vi "Generate Acoustic Sine Signal.vi"(0 "Sampling Rate":dbl, 1 "Maximum No. of Samples Allowed":i32=65536, 5 "Frequency":dbl, 7 "Sine wave amplitude":dbl=0.01 format="%#_13g", 11 "error in (no error)":errorcluster) -> (4 "waveform":waveform(dbl), 6 "Actual Frequency":dbl, 15 "error out":errorcluster)   [LabVIEW 2020]
doc: "Generate Acoustic Sine Signal VI checks whether the requested frequency can be produced for the given sample rate and outputs Whole Sine waveform of integral multiple of samples for rounded off Sine frequency."
uses:
  <vilib>/Analysis/NI_AALBase.lvlib
  <vilib>/gmath/NI_Gmath.lvlib
  <vilib>/measure/NI_MABase.lvlib
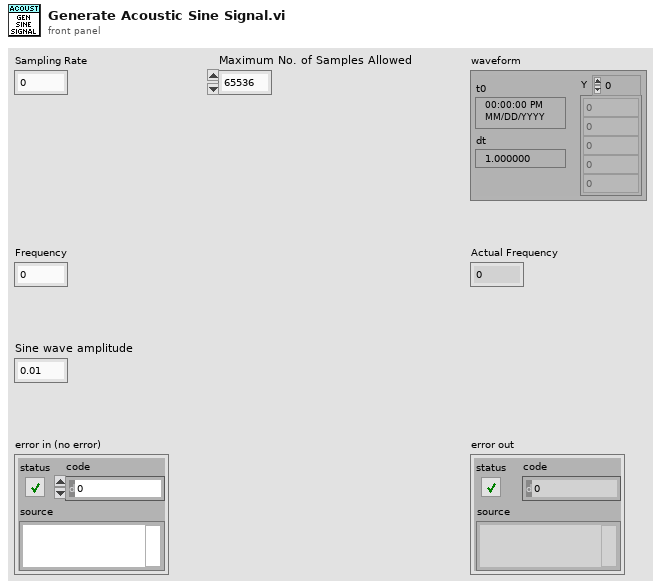
[diagram p1: front panel]
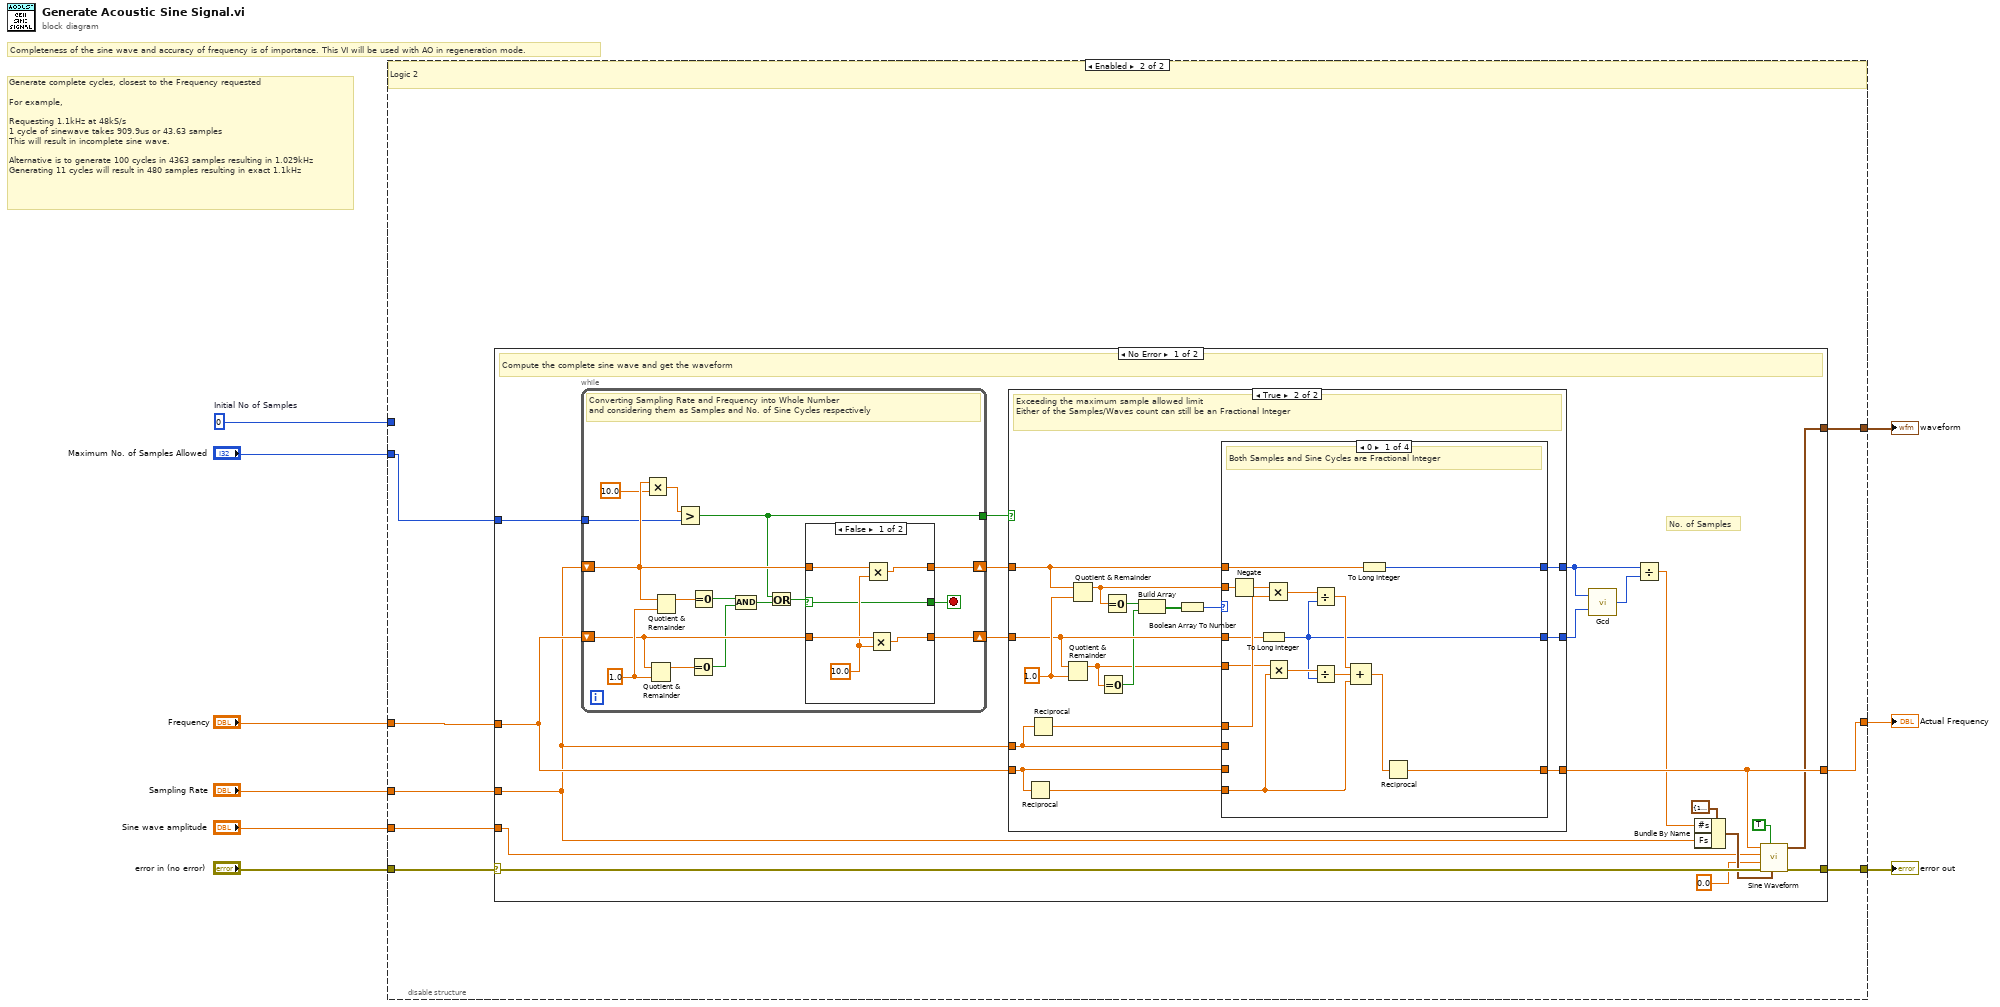
[diagram p0: block diagram]
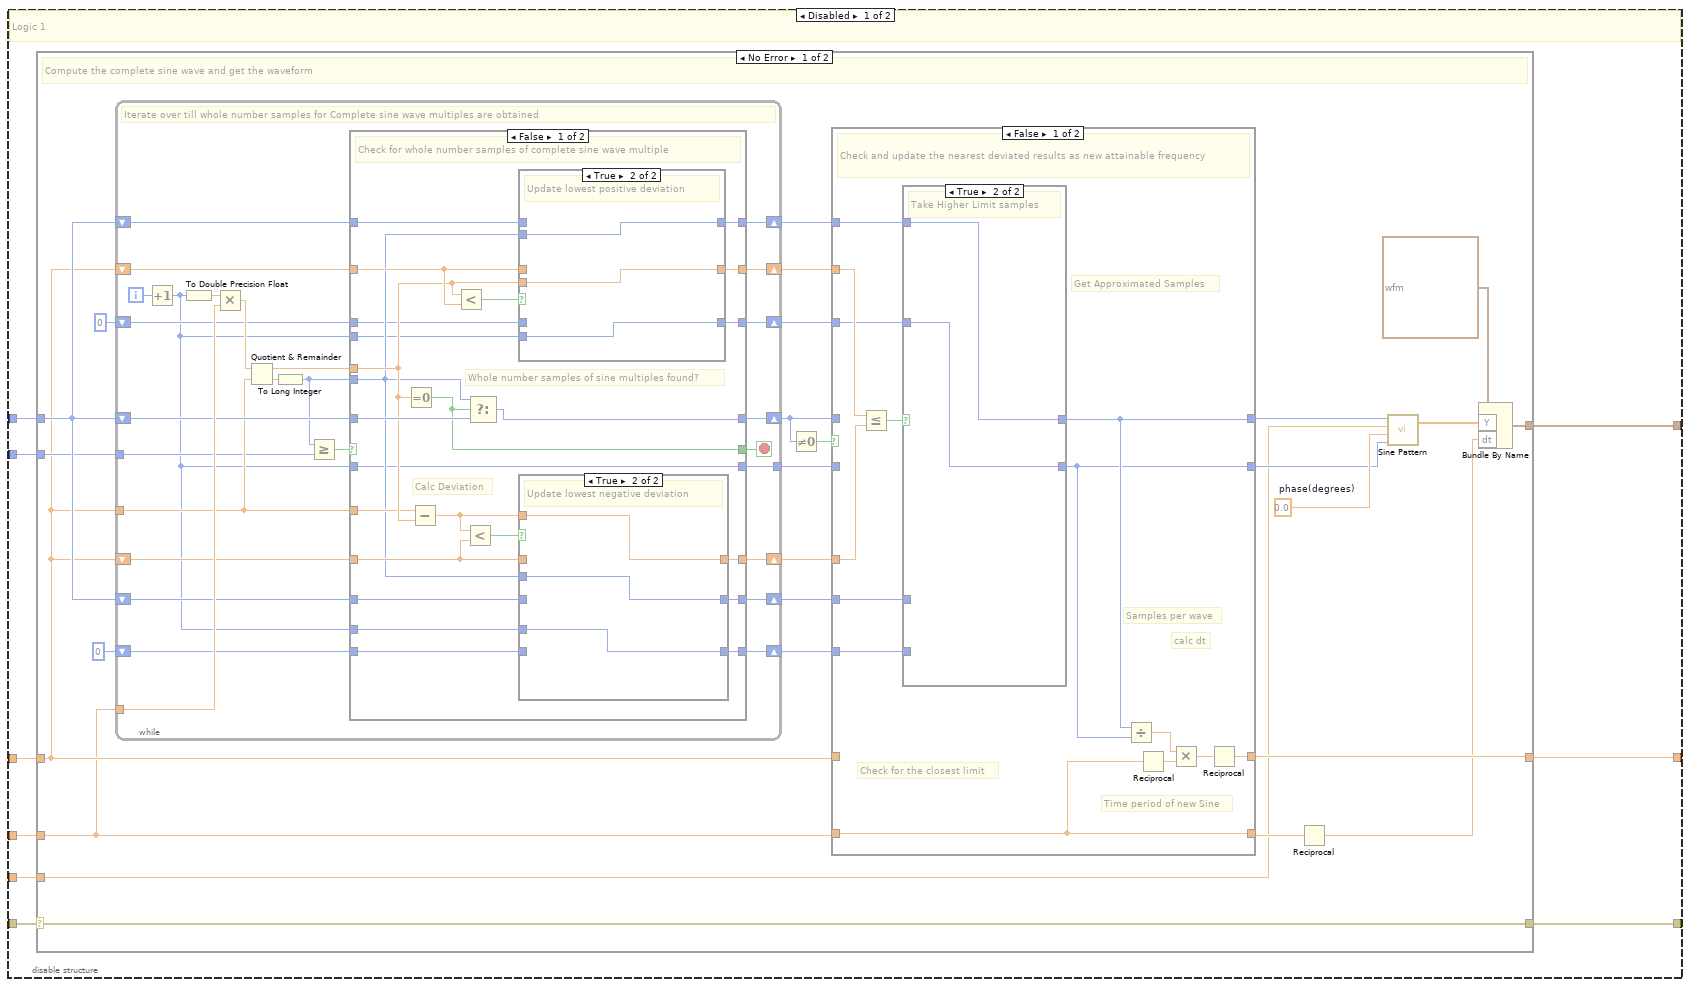
[diagram p2: hidden frame]
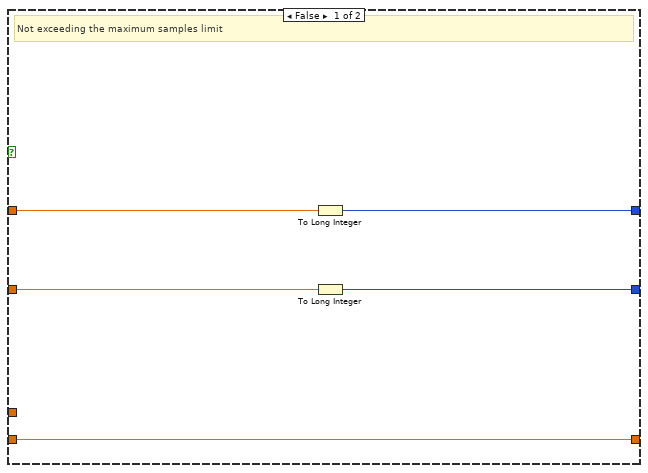
[diagram p9: hidden frame]
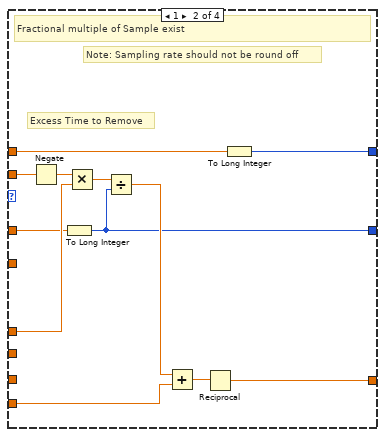
[diagram p10: hidden frame]
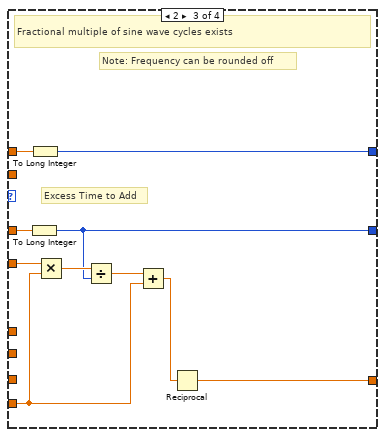
[diagram p11: hidden frame]
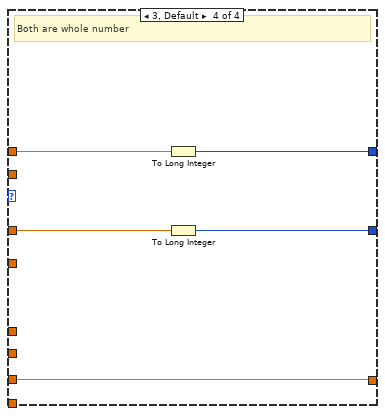
[diagram p12: hidden frame]
diagram:
  w9 = 0  # Initial No of Samples
  # "Completeness of the sine wave and accuracy of frequency is of importance. This VI will be used with AO in regeneration mode."
  # "Generate complete cycles, closest to the Frequency requested\n\nFor example,\n\nRequesting 1.1kHz at 48kS/s\n1 cycle of sinewave takes 909.9us or 43.63 samples\nThis will result in incomplete sine wave. \n\nAlternative is to generate 100 cycles in 4363 samples resulting in 1.029kHz \nGenerating 11 cycles will result in 480 samples resulting in exact 1.1kHz"
  n1 = disable-structure shown="Enabled" {
    disable-tunnel: w9 -> [w18 _]
    disable-tunnel: "Maximum No. of Samples Allowed" -> [w17 w147]
    disable-tunnel: "Frequency" -> [w16 w145]
    disable-tunnel: [w15 w141] -> w6
    disable-tunnel: "Sampling Rate" -> [w14 w146]
    disable-tunnel: [w13 w140] -> w4
    disable-tunnel: "error in (no error)" -> [w12 w144]
    disable-tunnel: [w11 w142] -> w2
    disable-tunnel: "Sine wave amplitude" -> [w10 w143]
    frame Disabled {
      # "Logic 1"
      n2 = case shown="No Error" w12 {
        selector: w12 -> [w25 w139]
        tunnel: w18 -> [w44 _]
        tunnel: w17 -> [w43 _]
        tunnel: w16 -> [w37 _]
        tunnel: [w36 _] -> w15
        tunnel: w14 -> [w35 _]
        tunnel: [w26 _] -> w13
        tunnel: [w25 w139] -> w11
        tunnel: w10 -> [w24 _]
        frame No Error {
          w32 = 0.0  # phase(degrees)
          # "Compute the complete sine wave and get the waveform"
          n3 = while {
            tunnel: w35 -> [w69]
            tunnel: w37 -> [w60]
            shift-right: [w65] -> w41
            shift-left: w44 -> [w64]
            shift-right: [w66] -> w39
            shift-left: w37 -> [w67]
            shift-right: [w62] -> w42
            shift-left: w44 -> [w63]
            shift-right: [w58] -> w38
            shift-left: w37 -> [w59]
            shift-right: [w56] -> w40
            shift-left: w44 -> [w57]
            tunnel: w43 -> [w55]
            tunnel: [w50] -> w34
            shift-right: [w49] -> w19
            shift-left: 0 -> [w48]
            shift-right: [w45] -> w20
            shift-left: 0 ("Initial No of Samples") -> [w47]
            i -> [w71]
            stop <- w51 stop-if-true
            # "Iterate over till whole number samples for Complete sine wave multiples are obtained"
            n4 = Increment(x=w71) -> (x+1=w46:i32)
            n5 = To Double Precision Float(number=w46) -> (double precision float=w70:dbl)
            n6 = Multiply(x=w70, y=w69) -> (x*y=w68:dbl)
            n7 = Quotient & Remainder(x=w68, y=w60) -> (x-y*floor(x/y)=w61:dbl, floor(x/y)=w54:dbl)
            n8 = To Long Integer(number=w54) -> (32bit integer=w53:i32)
            n9 = Greater Or Equal?(x=w53, y=w55) -> (x >= y?=w52:bool)
            n10 = case shown="False" w52 {
              selector: w52 -> [_ w116]
              tunnel: w67 -> [w94 w114]
              tunnel: [w93 w114] -> w66
              tunnel: [w92 w113] -> w65
              tunnel: w64 -> [w91 w113]
              tunnel: w63 -> [w90 w115]
              tunnel: [w89 w115] -> w62
              tunnel: w61 -> [w88 _]
              tunnel: w60 -> [w87 _]
              tunnel: w59 -> [w84 w112]
              tunnel: [w83 w112] -> w58
              tunnel: w57 -> [w82 w111]
              tunnel: [w81 w111] -> w56
              tunnel: w53 -> [w80 _]
              tunnel: [w78 w116] -> w51
              tunnel: w46 -> [w79 w110]
              tunnel: [w79 w110] -> w50
              tunnel: w46 -> [w77 _]
              tunnel: [w76 w109] -> w49
              tunnel: w48 -> [w75 w109]
              tunnel: w47 -> [w74 w108]
              tunnel: w46 -> [w72 _]
              tunnel: [w73 w108] -> w45
              frame False {
                # "Calc Deviation"
                # "Whole number samples of sine multiples found?"
                # "Check for whole number samples of complete sine wave multiple"
                n11 = Equal To 0?(x=w88) -> (x = 0?=w78:bool)
                n12 = Subtract(x=w87, y=w88) -> (x-y=w85:dbl)
                n13 = Less?(x=w88, y=w94) -> (x < y?=w95:bool)
                n14 = Less?(x=w85, y=w84) -> (x < y?=w86:bool)
                n15 = Select(t=w80, s=w78, f=w90) -> (s? t:f=w89:i32)
                n16 = case shown="True" w95 {
                  tunnel: w94 -> [w104 _]
                  tunnel: w88 -> [_ w107]
                  tunnel: [w104 w107] -> w93
                  tunnel: [w103 w106] -> w92
                  tunnel: w91 -> [w103 _]
                  tunnel: w80 -> [_ w106]
                  tunnel: w77 -> [_ w105]
                  tunnel: [w102 w105] -> w76
                  tunnel: w75 -> [w102 _]
                  frame False {
                    # "No Update"
                  }
                  frame True {
                    # "Update lowest positive deviation"
                  }
                }
                n17 = case shown="True" w86 {
                  tunnel: w85 -> [_ w101]
                  tunnel: w84 -> [w98 _]
                  tunnel: [w98 w101] -> w83
                  tunnel: w80 -> [_ w100]
                  tunnel: w82 -> [w97 _]
                  tunnel: [w97 w100] -> w81
                  tunnel: w74 -> [w96 _]
                  tunnel: [w96 w99] -> w73
                  tunnel: w72 -> [_ w99]
                  frame False {
                    # "No Update"
                  }
                  frame True {
                    # "Update lowest negative deviation"
                  }
                }
              }
              frame True {
                # "Maximum sample limit has been reached\nExit the Looping"
              }
            }
          }
          n18 = Not Equal To 0?(x=w42) -> (x != 0?=w23:bool)
          n19 = case shown="False" w23 {
            tunnel: w42 -> [_ w138]
            tunnel: w41 -> [w120 _]
            tunnel: w40 -> [w122 _]
            tunnel: [w118 w138] -> w33
            tunnel: w39 -> [w130 _]
            tunnel: w38 -> [w129 _]
            tunnel: w37 -> [_ w137]
            tunnel: [w126 w137] -> w36
            tunnel: w35 -> [w124 w135]
            tunnel: w34 -> [_ w136]
            tunnel: [w117 w136] -> w31
            tunnel: [w124 w135] -> w28
            tunnel: w20 -> [w121 _]
            tunnel: w19 -> [w119 _]
            frame False {
              # "Time period of new Sine"
              # "calc dt"
              # "Samples per wave"
              # "Get Approximated Samples"
              # "Check for the closest limit"
              # "Check and update the nearest deviated results as new attainable frequency"
              n20 = Less Or Equal?(x=w130, y=w129) -> (x <= y?=w123:bool)
              n21 = case shown="True" w123 {
                tunnel: w122 -> [w132 _]
                tunnel: w121 -> [w131 _]
                tunnel: w120 -> [_ w134]
                tunnel: w119 -> [_ w133]
                tunnel: [w132 w134] -> w118
                tunnel: [w131 w133] -> w117
                frame False {
                  # "Take Lower limit samples"
                }
                frame True {
                  # "Take Higher Limit samples"
                }
              }
              n22 = Divide(x=w118, y=w117) -> (x/y=w127:dbl)
              n23 = Reciprocal(x=w124) -> (1/x=w128:dbl)
              n24 = Multiply(x=w127, y=w128) -> (x*y=w125:dbl)
              n25 = Reciprocal(x=w125) -> (1/x=w126:dbl)
            }
            frame True {
              # "Whole number samples of complete sine wave multiples are found within the max samples range"
            }
          }
          n26 = Reciprocal(x=w28) -> (1/x=w27:dbl)
          n27 = call <vilib>:"Sine Pattern.vi"("cycles"=w31, "phase(degrees)"=w32, "amplitude"=w24, "samples"=w33) -> ("Sinusoidal Pattern"=w29:dbl[])  [unwired: 1 out]
          n28 = Bundle By Name(cluster=waveform(dbl) {"t0"=timestamp(0 s since 1904-01-01), "dt"=1.0, "Y"=[]} ("waveform"), "Y"=w29, "dt"=w27) -> (w26:waveform(dbl))
        }
        frame Error {
          # "Error scenario - Do Nothing"
        }
      }
    }
    frame Enabled {
      # "Logic 2"
      n29 = case shown="No Error" w144 {
        selector: w144 -> [w155 w255]
        tunnel: w145 -> [w159 _]
        tunnel: w146 -> [w156 _]
        tunnel: [w154 w255] -> w142
        tunnel: w143 -> [w152 _]
        tunnel: w147 -> [w165 _]
        tunnel: [w158 _] -> w141
        tunnel: [w148 _] -> w140
        frame No Error {
          # "No. of Samples"
          # "Compute the complete sine wave and get the waveform"
          n30 = while {
            shift-right: [w244] -> w163
            shift-left: w156 -> [w236]
            shift-right: [w242] -> w161
            shift-left: w159 -> [w243]
            tunnel: w165 -> [w234]
            tunnel: [w230] -> w164
            stop <- w237 stop-if-true
            w245 = 1.0 ("y")
            # "Converting Sampling Rate and Frequency into Whole Number\nand considering them as Samples and No. of Sine Cycles respectively"
            n31 = Multiply(x=w236, y=10.0) -> (x*y=w233:dbl)
            n32 = Quotient & Remainder(x=w243, y=w245) -> (x-y*floor(x/y)=w241:dbl)  [unwired: 1 out]
            n33 = Quotient & Remainder(x=w236, y=w245) -> (x-y*floor(x/y)=w240:dbl)  [unwired: 1 out]
            n34 = Greater?(x=w233, y=w234) -> (0:w230:bool)
            n35 = Equal To 0?(x=w241) -> (x = 0?=w238:bool)
            n36 = Equal To 0?(x=w240) -> (x = 0?=w239:bool)
            n37 = Compound Arithmetic op=AND(w239, w238) -> (w231:bool)
            n38 = Or(x=w230, y=w231) -> (x .or. y?=w232:bool)
            n39 = case shown="False" w232 {
              selector: w232 -> [w246 w252]
              tunnel: w236 -> [w251 w254]
              tunnel: [w247 w254] -> w244
              tunnel: w243 -> [w250 w253]
              tunnel: [w248 w253] -> w242
              tunnel: [w246 w252] -> w237
              frame False {
                w249 = 10.0 ("y")
                n40 = Multiply(x=w251, y=w249) -> (x*y=w247:dbl)
                n41 = Multiply(x=w250, y=w249) -> (x*y=w248:dbl)
              }
              frame True {
              }
            }
          }
          n42 = case shown="True" w164 {
            tunnel: w163 -> [w171 w184]
            tunnel: [w170 w187] -> w162
            tunnel: w161 -> [w169 w183]
            tunnel: [w168 w186] -> w160
            tunnel: w156 -> [_ w173]
            tunnel: w159 -> [w167 w174]
            tunnel: [w167 w175] -> w158
            frame False {
              # "Not exceeding the maximum samples limit"
              n43 = To Long Integer(number=w171) -> (32bit integer=w170:i32)
              n44 = To Long Integer(number=w169) -> (32bit integer=w168:i32)
            }
            frame True {
              w185 = 1.0 ("y")
              # "Exceeding the maximum sample allowed limit\nEither of the Samples/Waves count can still be an Fractional Integer"
              n45 = Reciprocal(x=w174) -> (1/x=w176:dbl)
              n46 = Reciprocal(x=w173) -> (1/x=w177:dbl)
              n47 = Quotient & Remainder(x=w183, y=w185) -> (x-y*floor(x/y)=w172:dbl)  [unwired: 1 out]
              n48 = Quotient & Remainder(x=w184, y=w185) -> (x-y*floor(x/y)=w178:dbl)  [unwired: 1 out]
              n49 = Equal To 0?(x=w172) -> (x = 0?=w181:bool)
              n50 = Equal To 0?(x=w178) -> (x = 0?=w182:bool)
              n51 = Build Array(w182, w181) -> (w180:bool[])
              n52 = Boolean Array To Number(Boolean array=w180) -> (number=w179:u32)
              n53 = case shown="0" w179 {
                tunnel: [w197 w210 w223 w227] -> w187
                tunnel: [w188 w203 w215 w226] -> w186
                tunnel: w184 -> [w198 w208 w224 w229]
                tunnel: w183 -> [w194 w206 w216 w228]
                tunnel: w178 -> [w202 w205 _ _]
                tunnel: w177 -> [w201 w214 _ _]
                tunnel: w176 -> [w190 w213 w220 _]
                tunnel: [w199 w211 w219 w225] -> w175
                tunnel: w174 -> [_ _ _ w225]
                tunnel: w173 -> [_ _ _ _]
                tunnel: w172 -> [w191 _ w221 _]
                frame 0 {
                  # "Both Samples and Sine Cycles are Fractional Integer"
                  n54 = Negate(x=w202) -> (-x=w196:dbl)
                  n55 = To Long Integer(number=w194) -> (32bit integer=w188:i32)
                  n56 = Multiply(x=w196, y=w201) -> (x*y=w195:dbl)
                  n57 = Multiply(x=w191, y=w190) -> (x*y=w192:dbl)
                  n58 = Divide(x=w195, y=w188) -> (x/y=w193:dbl)
                  n59 = Divide(x=w192, y=w188) -> (x/y=w189:dbl)
                  n60 = Compound Arithmetic op=ADD(w193, w189, w190) -> (w200:dbl)
                  n61 = To Long Integer(number=w198) -> (32bit integer=w197:i32)
                  n62 = Reciprocal(x=w200) -> (1/x=w199:dbl)
                }
                frame 1 {
                  # "Excess Time to Remove"
                  # "Note: Sampling rate should not be round off"
                  # "Fractional multiple of Sample exist"
                  n63 = Negate(x=w205) -> (-x=w204:dbl)
                  n64 = To Long Integer(number=w206) -> (32bit integer=w203:i32)
                  n65 = Multiply(x=w204, y=w214) -> (x*y=w209:dbl)
                  n66 = Divide(x=w209, y=w203) -> (x/y=w207:dbl)
                  n67 = Add(x=w207, y=w213) -> (x+y=w212:dbl)
                  n68 = Reciprocal(x=w212) -> (1/x=w211:dbl)
                  n69 = To Long Integer(number=w208) -> (32bit integer=w210:i32)
                }
                frame 2 {
                  # "Excess Time to Add"
                  # "Note: Frequency can be rounded off"
                  # "Fractional multiple of sine wave cycles exists"
                  n70 = To Long Integer(number=w216) -> (32bit integer=w215:i32)
                  n71 = To Long Integer(number=w224) -> (32bit integer=w223:i32)
                  n72 = Multiply(x=w221, y=w220) -> (x*y=w218:dbl)
                  n73 = Divide(x=w218, y=w215) -> (x/y=w217:dbl)
                  n74 = Add(x=w217, y=w220) -> (x+y=w222:dbl)
                  n75 = Reciprocal(x=w222) -> (1/x=w219:dbl)
                }
                frame 3, Default {
                  # "Both are whole number"
                  n76 = To Long Integer(number=w229) -> (32bit integer=w227:i32)
                  n77 = To Long Integer(number=w228) -> (32bit integer=w226:i32)
                }
              }
            }
          }
          n78 = call <vilib>:"Gcd.vi"("y"=w160, "x"=w162) -> ("gcd(x,y)"=w166:i32)
          n79 = Divide(x=w162, y=w166) -> (x/y=w150:dbl)
          n80 = Bundle By Name(cluster=cluster{"Fs":dbl, "#s":dbl} {"Fs"=1000.0, "#s"=1000.0} ("sampling info"), "#s"=w150, "Fs"=w156) -> (w153:cluster{"Fs":dbl, "#s":dbl})
          n81 = call <vilib>:"Sine Waveform.vi"("sampling info"=w153, "reset signal"=TRUE, "error in (no error)"=w155, "phase"=0.0, "amplitude"=w152, "frequency"=w158) -> ("error out"=w154:errorcluster, "signal out"=w148:waveform(dbl))  [unwired: 4 in]
        }
        frame Error {
          # "Error scenario - Do Nothing"
        }
      }
    }
  }
  "error out" <- w2
  "waveform" <- w4
  "Actual Frequency" <- w6
